vi "QueueManagerGV.vi"(7 "Command":enum16{"Get", "Set Logging", "Set Queue"}(ring), 10 "Logging":bool, 11 "Queue in":refnum<queue>) -> (2 "Logging":bool, 3 "Queue":refnum<queue>)   [LabVIEW 2017]
uses:
  Type Defs/telemetryReading.ctl
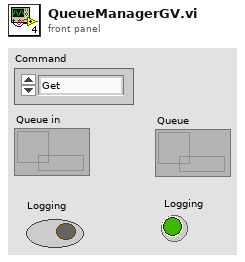
[diagram p1: front panel]
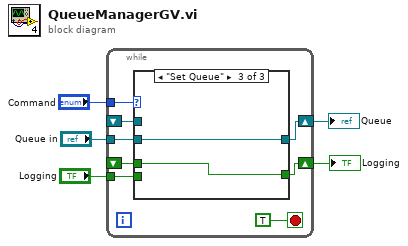
[diagram p0: block diagram]
diagram:
  n1 = while {
    tunnel: "Command" -> [w13]
    tunnel: "Queue in" -> [w10]
    shift-right: [w11] -> w3
    shift-left: _ -> [w9]
    tunnel: "Logging" -> [w8]
    shift-right: [w7] -> w1
    shift-left: _ -> [w6]
    stop <- TRUE stop-if-true
    n2 = case shown="\"Set Queue\"" w13 {
      tunnel: [w15 w16 w19] -> w11
      tunnel: w10 -> [_ _ w19]
      tunnel: w9 -> [w15 w16 _]
      tunnel: [w14 w17 w18] -> w7
      tunnel: w8 -> [_ w17 _]
      tunnel: w6 -> [w14 _ w18]
      frame "Get", Default {
      }
      frame "Set Logging" {
      }
      frame "Set Queue" {
      }
    }
  }
  "Queue" <- w3
  "Logging" <- w1
